vi "evaluate.vi"(8 "error in (no error)":errorcluster, 10 "Point":dbl[](array[numeric]), 11 "Objective in":refnum<class "Objective.lvclass">) -> (0 "error out":errorcluster, 2 "Evaluation":dbl, 3 "Objective out":refnum<class "Objective.lvclass">)   [LabVIEW 2023, in "Objective.lvclass"]
uses:
  Objective.lvclass
  <vilib>/Analysis/_algsub.llb/Real Vector Norm.vi
  <vilib>/Analysis/NI_AALPro.lvlib
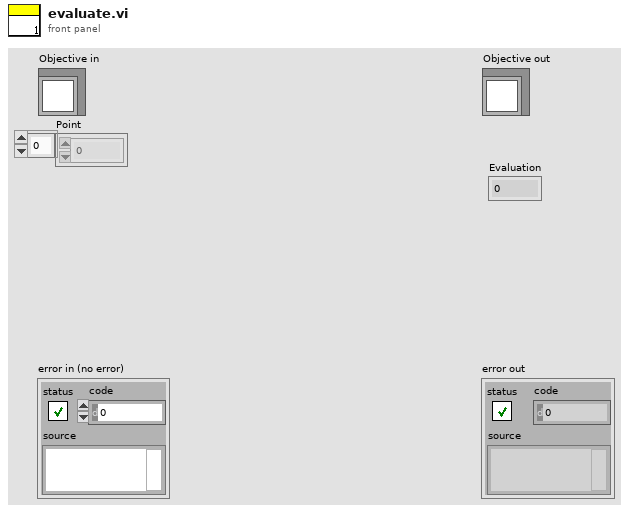
[diagram p1: front panel]
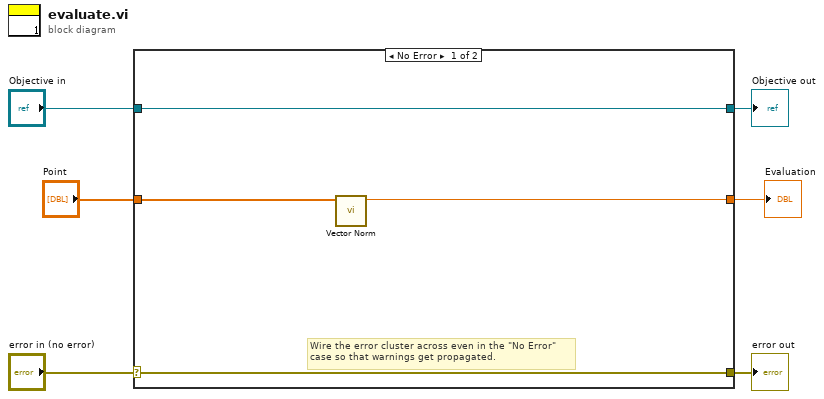
[diagram p0: block diagram]
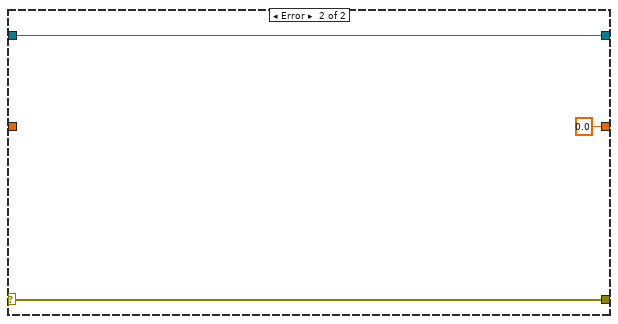
[diagram p2: hidden frame]
diagram:
  n1 = case shown="No Error" "error in (no error)" {
    selector: "error in (no error)" -> [w9 w13]
    tunnel: [w9 w13] -> w5
    tunnel: [w10 w12] -> w3
    tunnel: "Objective in" -> [w10 w12]
    tunnel: [w7 0.0 ("Evaluation")] -> w2
    tunnel: "Point" -> [w8 _]
    frame No Error {
      # "Wire the error cluster across even in the \"No Error\"\ncase so that warnings get propagated."
      n2 = call-poly <vilib>:"Vector Norm.vi"("Input Vector"=w8) -> ("norm"=w7:dbl)  [unwired: 9 in, 1 out]
    }
    frame Error {
    }
  }
  "error out" <- w5
  "Objective out" <- w3
  "Evaluation" <- w2
